vi "Temp to Volts.vi"() -> ()   [LabVIEW 2021]
panel:
  out "Voltage":sgl
  in  "Temperature":sgl
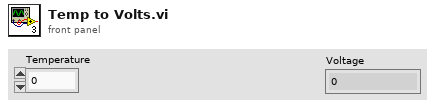
[diagram p1: front panel]
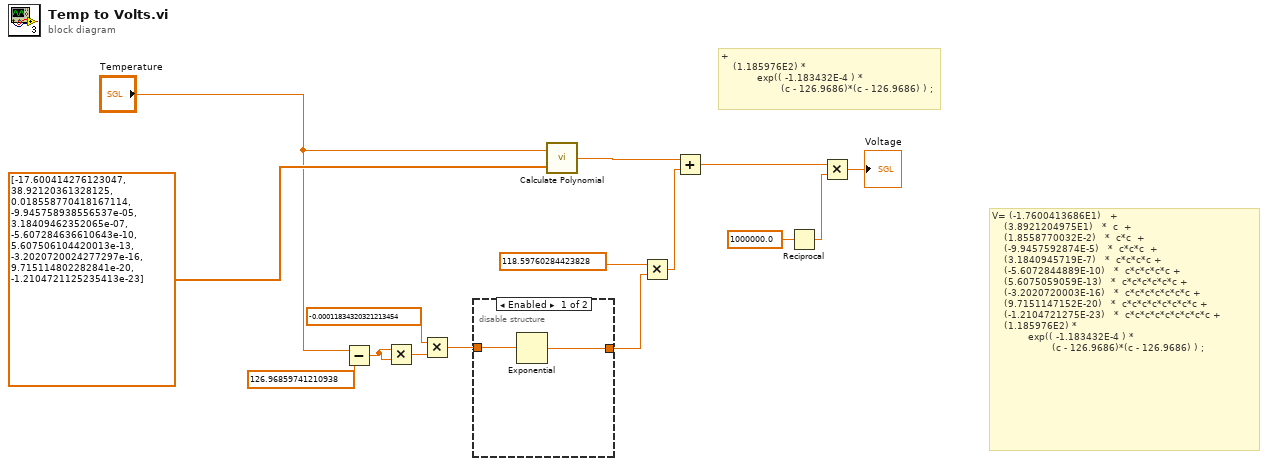
[diagram p0: block diagram]
diagram:
  # "+\n    (1.185976E2) * \n            exp(( -1.183432E-4 ) * \n                    (c - 126.9686)*(c - 126.9686) ) ;"
  # "V= (-1.7600413686E1)   +\n    (3.8921204975E1)   *  c  +\n    (1.8558770032E-2)   *  c*c  +\n    (-9.9457592874E-5)   *  c*c*c  +\n    (3.1840945719E-7)   *  c*c*c*c +\n    (-5.6072844889E-10)   *  c*c*c*c*c +\n    (5.6075059059E-13)   *  c*c*c*c*c*c +\n    (-3.2020720003E-16)   *  c*c*c*c*c*c*c +\n    (9.7151147152E-20)   *  c*c*c*c*c*c*c*c +\n    (-1.2104721275E-23)   *  c*c*c*c*c*c*c*c*c +\n    (1.185976E2) * \n            exp(( -1.183432E-4 ) * \n                    (c - 126.9686)*(c - 126.9686) ) ;"
  n1 = Subtract(x="Temperature", y=sgl 126.9686) -> (x-y=w11:sgl)
  n2 = Multiply(x=w11, y=w11) -> (x*y=w10:sgl)
  n3 = Multiply(x=sgl -0.0001183432, y=w10) -> (x*y=w6:sgl)
  n4 = disable-structure shown="Enabled" {
    disable-tunnel: w6 -> [w17 _]
    disable-tunnel: [w16 _] -> w5
    frame Enabled {
      n5 = Exponential(1:w17) -> (0:w16:sgl)
    }
    frame Disabled {
    }
  }
  n6 = call "Calculate Polynomial.vi"("Coefficients"=sgl[] [-17.600414, 38.921204, 0.01855877, -9.945759e-05, 3.1840946e-07, -5.6072846e-10, 5.607506e-13, -3.202072e-16, 9.715115e-20, -1.2104721e-23], "Value"="Temperature") -> ("Result"=w14:sgl)
  n7 = Multiply(x=sgl 118.5976, y=w5) -> (x*y=w7:sgl)
  n8 = Add(x=w14, y=w7) -> (x+y=w4:sgl)
  n9 = Reciprocal(x=sgl 1000000.0) -> (1/x=w1:sgl)
  n10 = Multiply(x=w4, y=w1) -> (x*y=→"Voltage":sgl)
